vi "TestConnection.vi"(8 "error in (no error)":errorcluster, 11 "ID In":i32) -> (0 "error out":errorcluster, 2 "code":i32, 3 "ID Out":i32)   [LabVIEW 2022 SP3, in "EClib functions.lvlib"]
uses:
  EClib functions.lvlib
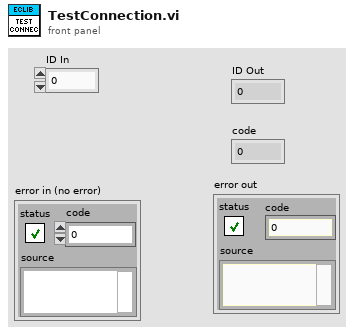
[diagram p1: front panel]
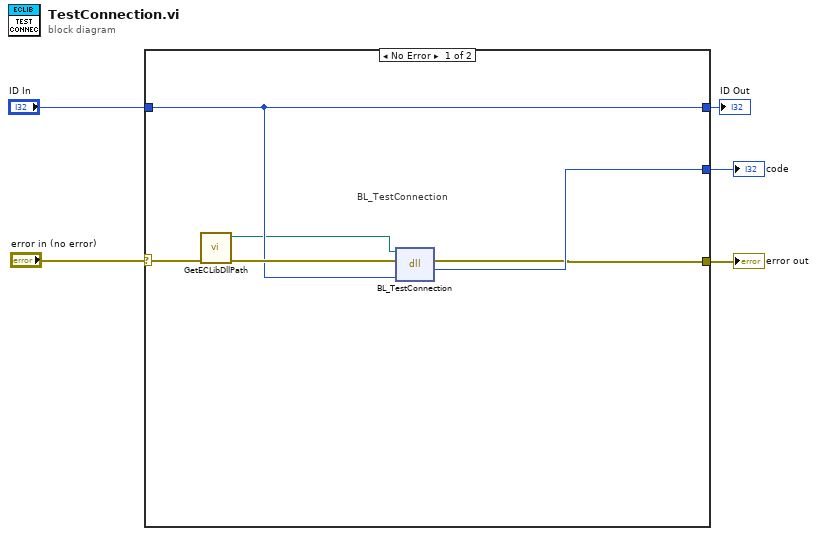
[diagram p0: block diagram]
diagram:
  n1 = case shown="No Error" "error in (no error)" {
    selector: "error in (no error)" -> [w11 w12]
    tunnel: [w7 w12] -> w2
    tunnel: "ID In" -> [w9 w13]
    tunnel: [w9 w13] -> w5
    tunnel: [w8 _] -> w1
    frame No Error {
      # "BL_TestConnection"
      n2 = call "GetECLibDllPath.vi"("error in (no error)"=w11) -> ("error out"=w10:errorcluster, "ECLibDLLPath"=w6:path)  [unwired: 9 in]
      n3 = dll-call lib="C:/EC-Lab Development Package/EC-Lab Development Package/EClib.dll" fn="BL_TestConnection"(path in=w6, error in=w10, "arg1"=w9) -> (error out=w7:errorcluster, "return type"=w8:i32)  [unwired: 2 in, 1 out]
    }
    frame Error {
    }
  }
  "error out" <- w2
  "ID Out" <- w5
  "code" <- w1
